vi "test_CD mockup (inline).vi"() -> ()   [LabVIEW 2020]
uses:
  <instrlib>/BTICardLib/Private/Initialize By Card Number and Core Number.vi
  <instrlib>/BTI1553Lib/Private/Channel/Configure/Configure All From XML.vi
  <instrlib>/BTICardLib/BTICardLV.lvlib
  <instrlib>/BTI1553Lib/BTI1553LV.lvlib
panel:
  out "Product String":string
  out "Card Type":string
  out "bytes read":i32
  out "channel count out":i32
  in  "channel handle array size in":i32=1
  out "XML load time ms":u32
  in  "card number":i32=1
  in  "core number":i32
  in  "configuration file path":path=path "c:/ni-rt/VeriStand/Custom Devices/Ballard - 1553/Board_1__Core_0__.xml"
  out "error out":errorcluster
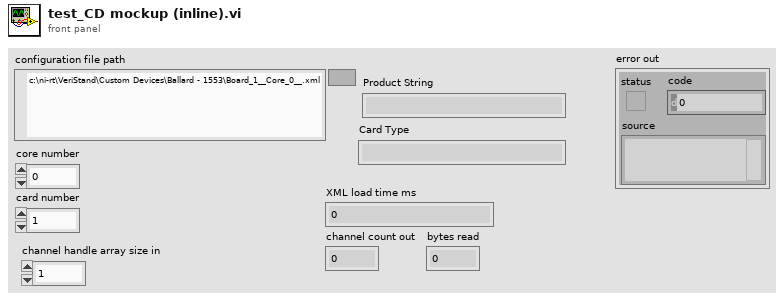
[diagram p1: front panel]
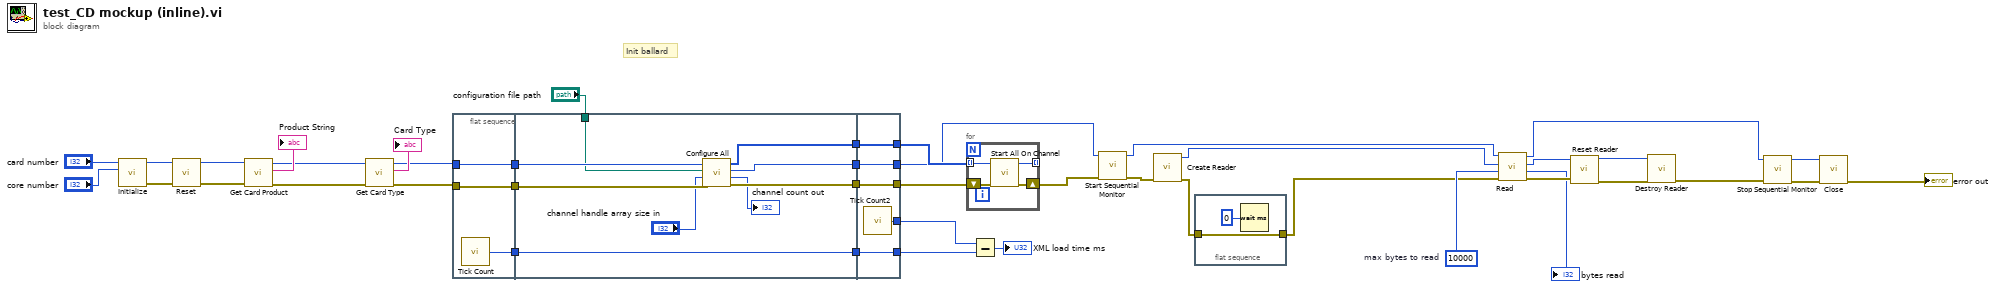
[diagram p0: block diagram]
diagram:
  w21 = 10000  # max bytes to read
  # "Init ballard"
  n1 = call-poly <instrlib>:"Initialize.vi"("core number"="core number", "card number"="card number") -> ("error out"=w43:errorcluster, "core handle out"=w42:u64)  [unwired: 8 in]
  n2 = call <instrlib>:"Reset.vi"("error in (no error)"=w43, "core handle in"=w42) -> ("error out"=w5:errorcluster, "core handle out"=w6:u64)  [unwired: 8 in]
  n3 = call <instrlib>:"Get Card Product.vi"("error in (no error)"=w5, "core handle in"=w6) -> ("error out"=w8:errorcluster, "product string out"=→"Product String":string, "core handle out"=w7:u64)  [unwired: 7 in]
  n4 = call <instrlib>:"Get Card Type.vi"("error in (no error)"=w8, "core handle in"=w7) -> ("error out"=w4:errorcluster, "type string out"=→"Card Type":string, "core handle out"=w3:u64)  [unwired: 7 in]
  n5 = flat-sequence {
    tunnel: w4 -> [w45]
    tunnel: w3 -> [w46]
    tunnel: [w46] -> w36
    tunnel: [w45] -> w35
    tunnel: [w44] -> w31
    tunnel: [w53] -> w38
    tunnel: [w52] -> w37
    tunnel: w36 -> [w55]
    tunnel: w35 -> [w54]
    tunnel: [w51] -> w32
    tunnel: w31 -> [w51]
    tunnel: "configuration file path" -> [w50]
    tunnel: [w49] -> w28
    tunnel: [w59] -> w27
    tunnel: [w60] -> w25
    tunnel: w38 -> [w60]
    tunnel: w37 -> [w59]
    tunnel: [w58] -> w34
    tunnel: [w57] -> w33
    tunnel: w32 -> [w57]
    tunnel: [w56] -> w26
    tunnel: w28 -> [w56]
    frame #0 {
      n6 = call "Tick Count"() -> ("Tick Count(mSec)"=w44:u32)
    }
    frame #1 {
      n7 = call-poly <instrlib>:"Configure All.vi"("error in (no error)"=w54, "channel handle array size in"="channel handle array size in", "configuration file path"=w50, "core handle in"=w55) -> ("error out"=w52:errorcluster, "channel count out"=→"channel count out":i32, "core handle out"=w53:u64, "channel handles out"=w49:u64[])  [unwired: 4 in]
    }
    frame #2 {
      n8 = call "Tick Count2"() -> ("Tick Count(mSec)"=w58:u32)
    }
  }
  n9 = for {
    shift-right: [w63] -> w24
    shift-left: w27 -> [w64]
    tunnel: w26 -> [w62] mode=indexing
    tunnel: [w61] -> _ mode=indexing
    n10 = call <instrlib>:"Start All On Channel.vi"("error in (no error)"=w64, "channel handle in"=w62) -> ("error out"=w63:errorcluster, "channel handle out"=w61:u64)  [unwired: 8 in]
  }
  n11 = Subtract(x=w34, y=w33) -> (x-y=→"XML load time ms":u32)
  n12 = call <instrlib>:"Start Sequential Monitor.vi"("error in (no error)"=w24, "core handle in"=w25) -> ("error out"=w23:errorcluster, "core handle out"=w22:u64)  [unwired: 8 in]
  n13 = call <instrlib>:"Create Reader.vi"("error in (no error)"=w23) -> ("error out"=w1:errorcluster, "core reader handle out"=w20:u64)  [unwired: 9 in]
  n14 = flat-sequence {
    tunnel: [w66] -> w2
    tunnel: w1 -> [w66]
    frame #0 {
      n15 = Wait (ms)(milliseconds to wait=u32 0) -> ()  [unwired: 1 out]
    }
  }
  n16 = call <instrlib>:"Read.vi"("error in (no error)"=w2, "max bytes to read"=w21, "core reader handle in"=w20, "core handle in"=w22) -> ("error out"=w16:errorcluster, "bytes read"=→"bytes read":i32, "core reader handle out"=w14:u64, "core handle out"=w13:u64)  [unwired: 4 in]
  n17 = call <instrlib>:"Reset Reader.vi"("error in (no error)"=w16, "reader handle in"=w14) -> ("error out"=w17:errorcluster, "reader handle out"=w19:u64)  [unwired: 8 in]
  n18 = call <instrlib>:"Destroy Reader.vi"("error in (no error)"=w17, "reader handle in"=w19) -> ("error out"=w18:errorcluster)  [unwired: 9 in]
  n19 = call <instrlib>:"Stop Sequential Monitor.vi"("error in (no error)"=w18, "core handle in"=w13) -> ("error out"=w11:errorcluster, "core handle out"=w12:u64)  [unwired: 8 in]
  n20 = call <instrlib>:"Close.vi"("error in (no error)"=w11, "core handle in"=w12) -> ("error out"=→"error out":errorcluster)  [unwired: 8 in, 1 out]
